vi "Set_Data.vi"(8 "error in (no error)":errorcluster caption="entrée d'erreur (pas d'erreur)", 11 "Firebase Benches en entrée":refnum<class "Firebase Packaging.lvclass">) -> (0 "error out":errorcluster caption="sortie d'erreur", 3 "Firebase Benches en sortie":refnum<class "Firebase Packaging.lvclass">)   [LabVIEW 2020, in "Library Instrument & Equipement.lvlib" / "Library FireBase.lvlib" / "Firebase Packaging.lvclass"]
doc: "Create New document\nPlease initialise the following values\n - Name BDD\n - Document\n - API Key"
uses:
  Firebase Packaging.lvclass
  C:/Users/ngarcin/OneDrive - Altyor/Standard TB/Class/Firebase/Source/Firebase Driver/Firebase Driver.lvclass
  Firebase Packaging.lvclass/Firebase Packaging.ctl
  Firebase Altyor/Firebase Altyor.lvclass
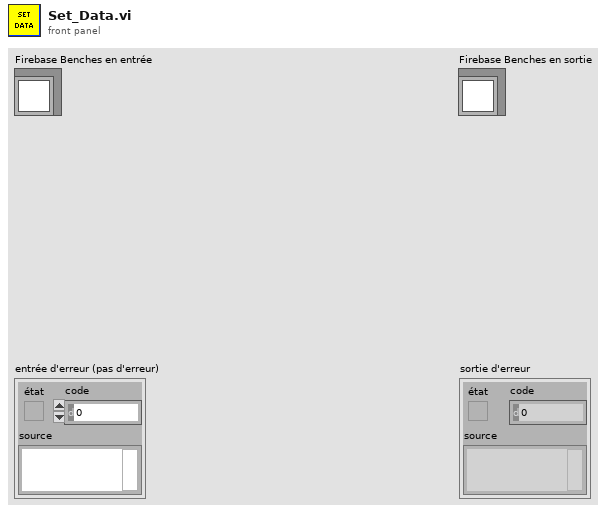
[diagram p1: front panel]
types:
  T1 = cluster{"fields":cluster{"Result":cluster{"booleanValue":bool}, "CreationDate":cluster{"timestampValue":string}, "Batch":cluster{"stringValue":string}, "SerialNumber":cluster{"stringValue":string}, "EndOfProduction":cluster{"timestampValue":string}, "PartNumber":cluster{"stringValue":string}, "OrderNumber":cluster{"stringValue":string}, "Operator":cluster{"stringValue":string}}}
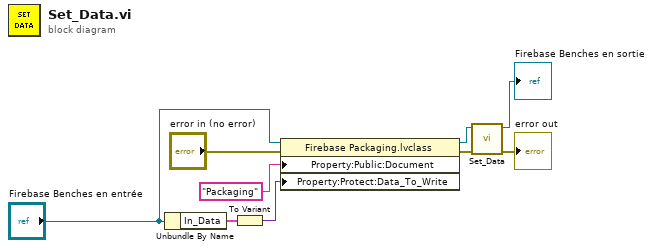
[diagram p0: block diagram]
diagram:
  n1 = Unbundle By Name("Firebase Benches en entrée") -> ("In_Data"=w3:T1)
  n2 = To Variant(anything=w3) -> (Variant=w2:variant)
  n3 = property class="Firebase Packaging.lvclass"(reference="Firebase Benches en entrée", error in="error in (no error)", "Property:Public:Document"="Packaging" ("Collection_to_find"), "Property:Protect:Data_To_Write"=w2) -> (reference out=w7:refnum<class "Firebase Packaging.lvclass">, error out=w6:errorcluster)
  n4 = call-parent "Set_Data.vi"("error in (no error)"=w6, "Firebase Altyor en entrée"=w7) -> ("error out"=→"error out":errorcluster, "Firebase Altyor en sortie"=→"Firebase Benches en sortie":refnum<class "Firebase Packaging.lvclass">)  [unwired: 8 in]
